vi "readTelemetryElevationData.vi"(8 "error in (no error)":errorcluster, 10 "Parser":refnum<class "U8ArrayParserAutoIndexing.lvclass">, 11 "M1M3SAL in":refnum<class "M1M3SAL.lvclass">) -> (0 "error out":errorcluster, 2 "EventSummaryState":variant, 3 "M1M3SAL out":refnum<class "M1M3SAL.lvclass">)   [LabVIEW 2016, in "M1M3SupportCommunicator.lvlib" / "M1M3SAL.lvclass"]
uses:
  M1M3SAL.lvclass
  Common_RT_Utilities/U8ArrayParserAutoIndexing/U8ArrayParserAutoIndexing.lvclass
  DataTypes/Topics/TelemetryElevationData.ctl
  DataTypes/Topics/Parts/Timestamp.ctl
  DataTypes/Topics/M1M3SupportTopics.lvlib
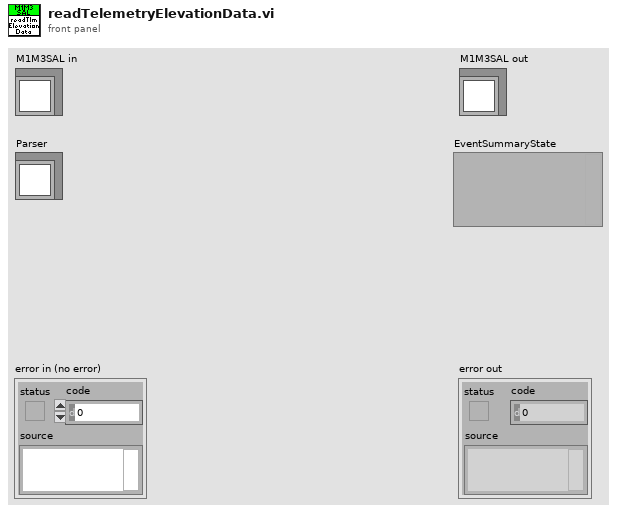
[diagram p1: front panel]
types:
  T1 = typedef "M1M3SupportTopics.lvlib/TelemetryElevationData.ctl" = cluster{"Timestamp":T2, "InclinometerElevation":dbl, "MeasuredElevation":dbl}
  T2 = typedef "M1M3SupportTopics.lvlib/Timestamp.ctl" = dbl
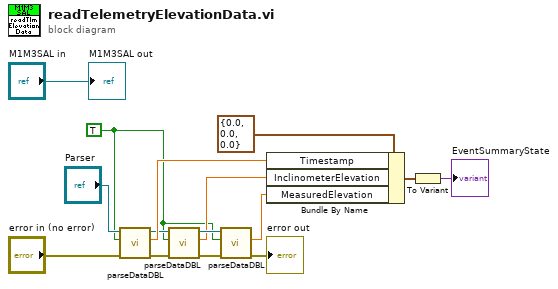
[diagram p0: block diagram]
diagram:
  w1 = TRUE ("OverrideSwapBytes")
  n1 = call "parseDataDBL.vi"("error in (no error)"="error in (no error)", "OverrideSwapBytes"=w1, "U8ArrayParserAutoIndexing in"="Parser") -> ("error out"=w7:errorcluster, "Data"=w10:dbl, "U8ArrayParserAutoIndexing out"=w9:refnum<class "U8ArrayParserAutoIndexing.lvclass">)  [unwired: 6 in]
  n2 = call "parseDataDBL.vi"("error in (no error)"=w7, "OverrideSwapBytes"=w1, "U8ArrayParserAutoIndexing in"=w9) -> ("error out"=w6:errorcluster, "Data"=w5:dbl, "U8ArrayParserAutoIndexing out"=w8:refnum<class "U8ArrayParserAutoIndexing.lvclass">)  [unwired: 6 in]
  n3 = call "parseDataDBL.vi"("error in (no error)"=w6, "OverrideSwapBytes"=w1, "U8ArrayParserAutoIndexing in"=w8) -> ("error out"=→"error out":errorcluster, "Data"=w4:dbl)  [unwired: 6 in, 1 out]
  n4 = Bundle By Name(cluster=T1 {"Timestamp"=0.0, "InclinometerElevation"=0.0, "MeasuredElevation"=0.0} ("TelemetryElevationData"), "Timestamp"=w10, "InclinometerElevation"=w5, "MeasuredElevation"=w4) -> (w14:T1)
  n5 = To Variant(anything=w14) -> (Variant=→"EventSummaryState":variant)
  "M1M3SAL out" <- "M1M3SAL in"
